vi "Create Output.vi"(8 "error in (no error)":errorcluster, 10 "Descriptor":string, 11 "output_actor in":refnum<class "Output Actor.lvclass">) -> (0 "error out":errorcluster, 3 "output_actor out":refnum<class "Output Actor.lvclass">)   [LabVIEW 2015, in "Output Actor.lvclass"]
uses:
  Output Actor.lvclass
  output/Output.lvclass
  Output Actor.lvclass/Output Actor.ctl
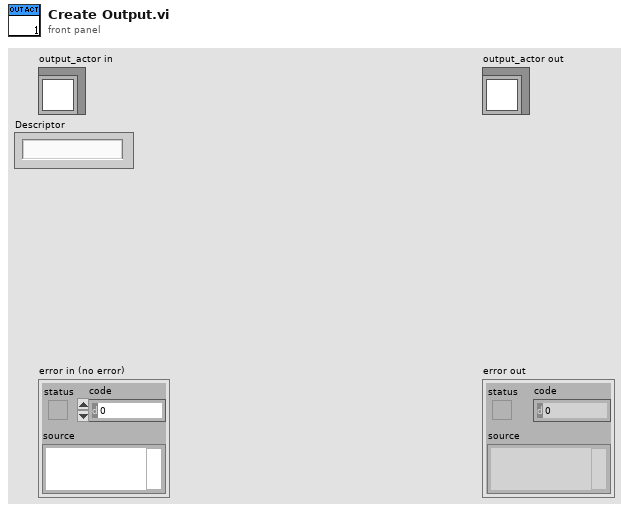
[diagram p1: front panel]
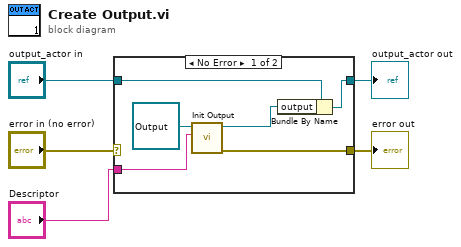
[diagram p0: block diagram]
diagram:
  n1 = case shown="No Error" "error in (no error)" {
    selector: "error in (no error)" -> [_ w13]
    tunnel: [w7 w13] -> w4
    tunnel: [w11 w12] -> w2
    tunnel: "output_actor in" -> [w8 w12]
    tunnel: "Descriptor" -> [w9 _]
    frame No Error {
      n2 = call "Init Output.vi"("Descriptor"=w9, "output in"=refnum<class "Output.lvclass"> refnum) -> ("error out"=w7:errorcluster, "output out"=w6:refnum<class "Output.lvclass">)  [unwired: 8 in]
      n3 = Bundle By Name(cluster=w8, "output"=w6) -> (w11:refnum<class "Output Actor.lvclass">)
    }
    frame Error {
    }
  }
  "error out" <- w4
  "output_actor out" <- w2
